vi "DigitalInput Example.vi"() -> ()   [LabVIEW 2012, in "Phidget Digital Input.lvlib"]
uses:
  <instrlib>/Phidgets/Phidget Digital Input/Phidget Digital Input.lvlib
  <instrlib>/Phidgets/Phidget Digital Input/Public/DigitalInputStart.vi
  <instrlib>/Phidgets/Phidget Digital Input/Public/DigitalInputClose.vi
  <instrlib>/Phidgets/Phidget Common/Phidget Common.lvlib
panel:
  in  "Is Hub Port?":bool
  out "State":bool
  out "error out":errorcluster
  in  "error in (no error)":errorcluster
  in  "Device Info":T1={"Serial Number"=-1, "Channel"=0, "Port"=0}
  out "Attached?":bool
  # "Yes"
  # "No"
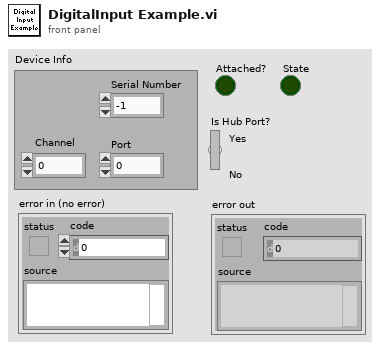
[diagram p1: front panel]
types:
  T1 = cluster{"Serial Number":i32, "Channel":i32, "Port":i32}
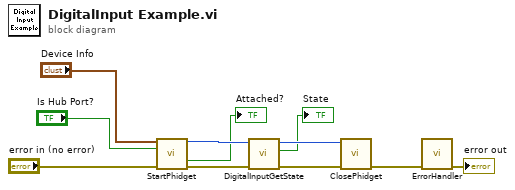
[diagram p0: block diagram]
diagram:
  n1 = call-poly <instrlib>:"StartPhidget.vi"("Device Info"="Device Info", "IsHubPort"="Is Hub Port?", "error in (no error)"="error in (no error)") -> ("Phidget ID"=w11:u64, "Attached?"=→"Attached?":bool, "error out"=w10:errorcluster)  [unwired: 9 in, 1 out]
  n2 = call <instrlib>:"DigitalInputGetState.vi"("error in (no error)"=w10, "Device In"=w11) -> ("error out"=w3:errorcluster, "State"=→"State":bool, "Device Out"=w4:u64)  [unwired: 5 in, 1 out]
  n3 = call-poly <instrlib>:"ClosePhidget.vi"("error in"=w3, "Device In"=w4) -> ("error out"=w6:errorcluster)  [unwired: 9 in]
  n4 = call <instrlib>:"ErrorHandler.vi"("error in"=w6) -> ("error out"=→"error out":errorcluster)  [unwired: 9 in, 1 out]
